vi "out of time.vi"(8 "error constant":errorcluster, 11 "DAQCascade512II 2":refnum<class "DAQCascade512II.lvclass">) -> (0 "error constant 2":errorcluster, 3 "DAQCascade512II":refnum<class "DAQCascade512II.lvclass">)   [LabVIEW 2012, in "DAQCascade512II.lvclass"]
uses:
  DAQCascade512II.lvclass
  DAQCascade512II.lvclass/DAQCascade512II.ctl
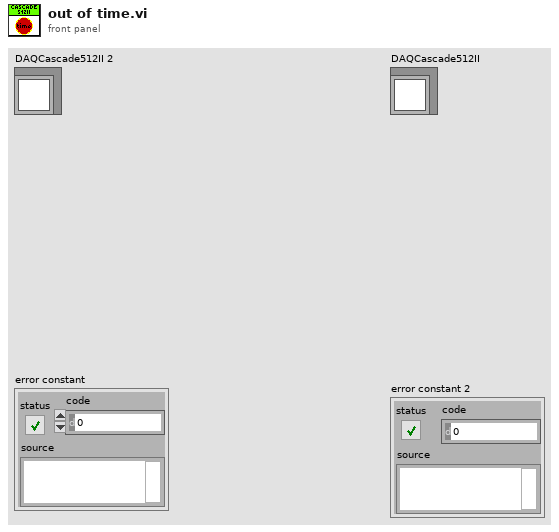
[diagram p1: front panel]
types:
  T1 = typedef "DAQCascade512II.lvclass/no. of frames.ctl" = u32
  T2 = typedef "DAQCascade512II.lvclass/Exposure (sec).ctl" = dbl
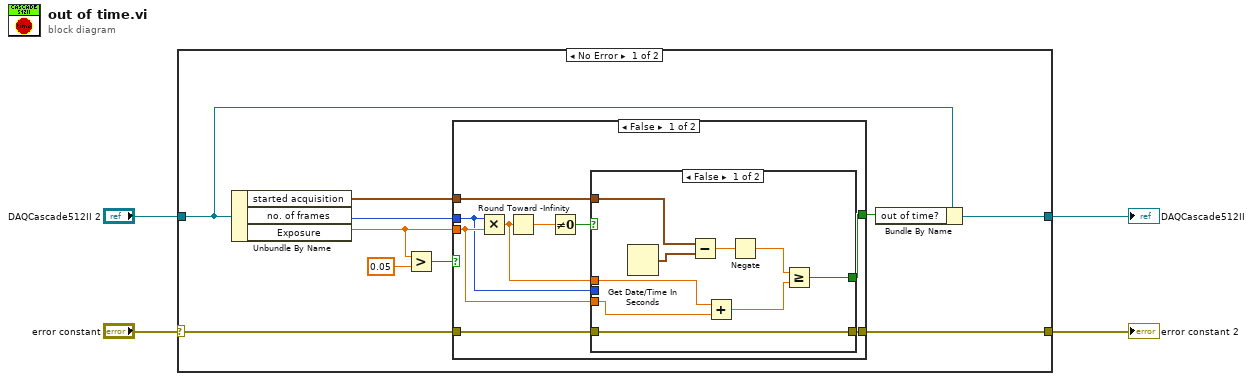
[diagram p0: block diagram]
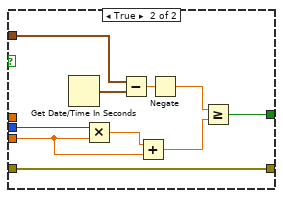
[diagram p2: hidden frame]
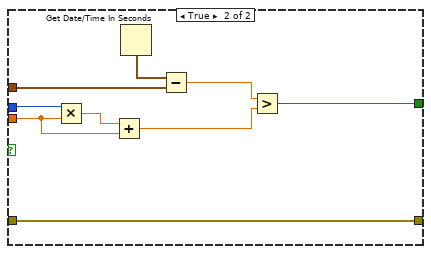
[diagram p3: hidden frame]
diagram:
  n1 = case shown="No Error" "error constant" {
    selector: "error constant" -> [w8 w52]
    tunnel: "DAQCascade512II 2" -> [w12 w53]
    tunnel: [w13 w52] -> w2
    tunnel: [w11 w53] -> w1
    frame No Error {
      n2 = Unbundle By Name(w12) -> ("started acquisition"=w14:timestamp, "no. of frames"=w10:T1, "Exposure"=w6:T2)
      n3 = Greater?(x=w6, y=0.05) -> (0:w7:bool)
      n4 = case shown="False" w7 {
        tunnel: w14 -> [w23 w50]
        tunnel: w8 -> [w22 w43]
        tunnel: [w21 w43] -> w13
        tunnel: w10 -> [w15 w49]
        tunnel: w6 -> [w20 w47]
        tunnel: [w18 w44] -> w9
        frame False {
          n5 = Multiply(x=w15, y=w20) -> (x*y=w16:T2)
          n6 = Round Toward -Infinity(1:w16) -> (0:w17:T2)
          n7 = Not Equal To 0?(x=w17) -> (x != 0?=w19:bool)
          n8 = case shown="False" w19 {
            tunnel: w16 -> [w26 _]
            tunnel: w23 -> [w30 w42]
            tunnel: [w29 w39] -> w21
            tunnel: w22 -> [w29 w39]
            tunnel: [w28 w36] -> w18
            tunnel: w20 -> [w24 w33]
            tunnel: w15 -> [_ w38]
            frame False {
              n9 = Get Date/Time In Seconds() -> (seconds since 1Jan1904=w31:timestamp)
              n10 = Subtract(x=w30, y=w31) -> (x-y=w32:dbl)
              n11 = Add(x=w26, y=w24) -> (x+y=w25:T2)
              n12 = Negate(x=w32) -> (-x=w27:dbl)
              n13 = Greater Or Equal?(x=w27, y=w25) -> (x >= y?=w28:bool)
            }
            frame True {
              n14 = Get Date/Time In Seconds() -> (seconds since 1Jan1904=w41:timestamp)
              n15 = Multiply(x=w38, y=w33) -> (x*y=w35:T2)
              n16 = Subtract(x=w42, y=w41) -> (x-y=w40:dbl)
              n17 = Add(x=w35, y=w33) -> (x+y=w34:T2)
              n18 = Negate(x=w40) -> (-x=w37:dbl)
              n19 = Greater Or Equal?(x=w37, y=w34) -> (x >= y?=w36:bool)
            }
          }
        }
        frame True {
          n20 = Multiply(x=w49, y=w47) -> (x*y=w48:T2)
          n21 = Add(x=w48, y=w47) -> (x+y=w45:T2)
          n22 = Get Date/Time In Seconds() -> (seconds since 1Jan1904=w51:timestamp)
          n23 = Subtract(x=w51, y=w50) -> (x-y=w46:dbl)
          n24 = Greater?(x=w46, y=w45) -> (0:w44:bool)
        }
      }
      n25 = Bundle By Name(cluster=w12, "out of time?"=w9) -> (w11:refnum<class "DAQCascade512II.lvclass">)
    }
    frame Error {
    }
  }
  "DAQCascade512II" <- w1
  "error constant 2" <- w2
